vi "controlCrosstalkThreshold.vi"(6 "SlipPhaseTime [us]":i32, 7 "Set":bool, 8 "error in":errorcluster, 9 "Threshold [nm]":i32, 10 "axis in":u8, 11 "connection ID":refnum<k5>) -> (0 "error out":errorcluster, 1 "Threshold out":i32, 2 "axis out":i32, 3 "connection ID":refnum<k5>, 4 "SlipPhaseTime out":i32)   [LabVIEW 2016]
doc: "This function retrieves or sets the threshold range and slip phase time which is used while moving another axis."
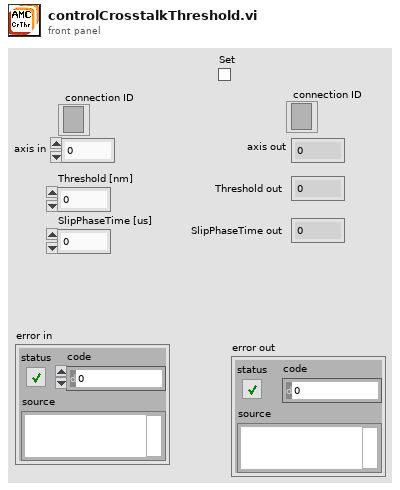
[diagram p1: front panel]
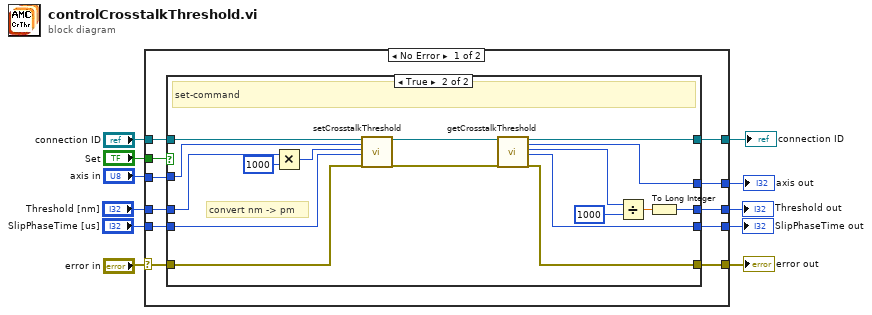
[diagram p0: block diagram]
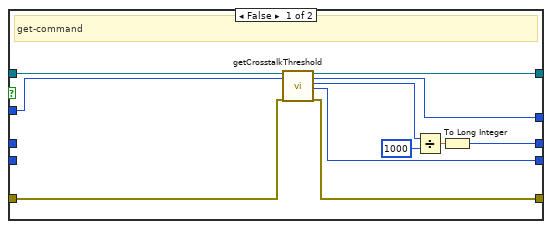
[diagram p2: hidden frame]
diagram:
  n1 = case shown="No Error" "error in" {
    selector: "error in" -> [w19 w55]
    tunnel: "axis in" -> [w22 w53]
    tunnel: [w14 w55] -> w10
    tunnel: "Set" -> [w20 _]
    tunnel: [w18 w54] -> w8
    tunnel: "connection ID" -> [w21 w54]
    tunnel: [w17 w53] -> w5
    tunnel: "Threshold [nm]" -> [w16 w52]
    tunnel: "SlipPhaseTime [us]" -> [w15 w51]
    tunnel: [w13 w52] -> w2
    tunnel: [w12 w51] -> w1
    frame No Error {
      n2 = case shown="True" w20 {
        tunnel: w21 -> [w33 w48]
        tunnel: w22 -> [w32 w46]
        tunnel: w19 -> [w31 w44]
        tunnel: [w29 w50] -> w18
        tunnel: [w28 w49] -> w17
        tunnel: w16 -> [_ w40]
        tunnel: w15 -> [_ w45]
        tunnel: [w30 w42] -> w14
        tunnel: [w23 w34] -> w13
        tunnel: [w27 w41] -> w12
        frame False {
          # "get-command"
          n3 = call "getCrosstalkThreshold.vi"("connection ID"=w33, "axis"=w32, "error in"=w31) -> ("connection ID"=w29:refnum<k5>, "axis_out"=w28:i32, "range"=w26:i32, "time"=w27:i32, "error out"=w30:errorcluster)  [unwired: 12 in]
          n4 = Divide(x=w26, y=1000) -> (x/y=w24:dbl)
          n5 = To Long Integer(number=w24) -> (32bit integer=w23:i32)
        }
        frame True {
          # "convert nm -> pm"
          # "set-command"
          n6 = Multiply(x=w40, y=1000) -> (x*y=w38:i32)
          n7 = call "setCrosstalkThreshold.vi"("connection ID"=w48, "axis"=w46, "threshold"=w38, "slipphasetime"=w45, "error in"=w44) -> ("connection ID"=w47:refnum<k5>, "error out"=w43:errorcluster)  [unwired: 12 in, 1 out]
          n8 = call "getCrosstalkThreshold.vi"("connection ID"=w47, "error in"=w43) -> ("connection ID"=w50:refnum<k5>, "axis_out"=w49:i32, "range"=w37:i32, "time"=w41:i32, "error out"=w42:errorcluster)  [unwired: 13 in]
          n9 = Divide(x=w37, y=1000) -> (x/y=w35:dbl)
          n10 = To Long Integer(number=w35) -> (32bit integer=w34:i32)
        }
      }
    }
    frame Error {
    }
  }
  "error out" <- w10
  "axis out" <- w5
  "connection ID" <- w8
  "Threshold out" <- w2
  "SlipPhaseTime out" <- w1
